vi "AB_Get_Skip_Close_Token.vi"(8 "error in":errorcluster) -> (0 "error out":errorcluster, 3 "Skip Close":bool)   [LabVIEW 2020]
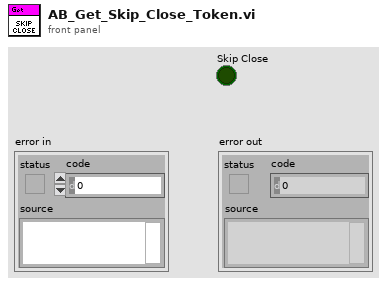
[diagram p1: front panel]
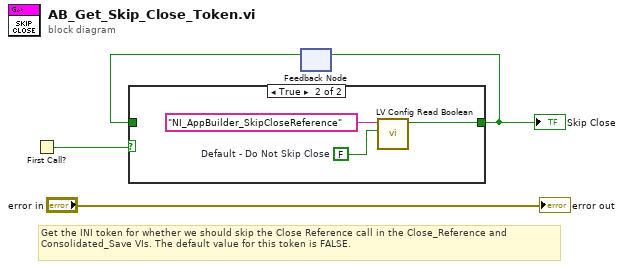
[diagram p0: block diagram]
diagram:
  # "Get the INI token for whether we should skip the Close Reference call in the Close_Reference and Consolidated_Save VIs. The default value for this token is FALSE."
  n1 = First Call?() -> (First Call?: T/F=w3:bool)
  n2 = feedback #1() -> (w1:bool)  [unwired: 1 in]
  n3 = case shown="True" w3 {
    tunnel: [w5 w8] -> w2
    tunnel: w1 -> [w5 _]
    frame False {
    }
    frame True {
      w6 = FALSE  # Default - Do Not Skip Close
      n4 = call <resource>:"LV Config Read Boolean.vi"("default value"=w6, "key"="NI_AppBuilder_SkipCloseReference") -> ("value"=w8:bool)  [unwired: 1 in, 4 out]
    }
  }
  "Skip Close" <- w2
  n5 = feedback-in #1(w2) -> ()
  "error out" <- "error in"
